vi "Climb.vi"(0 "Winch power":dbl=1.0, 1 "Toggle pistons":bool, 2 "Winch":bool, 3 "Unwinch":bool) -> ()   [LabVIEW 2019]
uses:
  <vilib>/Rock Robotics/WPI/Solenoid/WPI_SolenoidValue.ctl
  <vilib>/Rock Robotics/WPI/ThirdParty/Phoenix-LabVIEW/Motor Controller/Controls/CTRE_Phoenix_MotorControl_ControlMode.ctl
  <vilib>/functionblocks/FB Core/FB Core.xnode
  <vilib>/Rock Robotics/WPI/ThirdParty/Phoenix-LabVIEW/Motor Controller/Get/CTRE_Phoenix_MotorController_GetSupplyAndStatorCurrent_Enhanced.vi
  <vilib>/Rock Robotics/WPI/Solenoid/WPI_SolenoidSetEnum.vi
panel:
  out "Supply Current":dbl
  in  "Winch current threshold":dbl
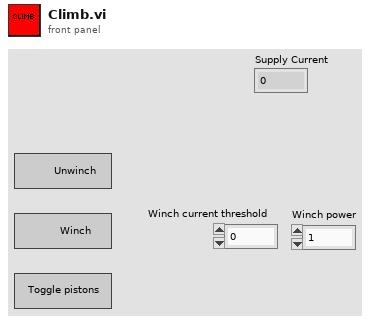
[diagram p1: front panel]
types:
  T1 = typedef "WPI_SolenoidValue.ctl" = enum16{"Off", "On", "Forward", "Reverse"}
  T2 = typedef "CTRE_Phoenix_MotorControl_ControlMode.ctl" = u16
  T3 = typedef "WPI_MotorControlDeviceRef.ctl" = cluster{"DeviceStatus":errorcluster, "Type":T4, "PWM":cluster{"PWM Channel":T5, "DeadBand":T6}, "CAN":cluster{"Device Number":u8, "SetOutput VI Ref":variant, "GetOutput VI Ref":variant, "Enable VI Ref":variant, "Disable VI Ref":variant, "Data":variant}, "Invert":bool, "DIO PWM":cluster{"PWM \"Enable\" Channel":T5, "DIOChannel":T7, "PWM Rate":dbl}}
  T4 = typedef "WPI_MotorControlType.ctl" = enum16{"PWM", "CAN", "DIO PWM"}
  T5 = typedef "FPGA_DIOPWMChannel.ctl" = enum8{"PWM 0", "PWM 1", "PWM 2", "PWM 3", "PWM 4", "PWM 5", "PWM 6", "PWM 7", "PWM 8", "PWM 9", "PWM MXP 0", "PWM MXP 1", "PWM MXP 2", "PWM MXP 3", "PWM MXP 4", "PWM MXP 5", "PWM MXP 6", "PWM MXP 7", "PWM MXP 8", "PWM MXP 9", "Invalid"}
  T6 = typedef "WPI_PWMDeadband.ctl" = cluster{"Name":string, "maxPositivePwm":i32, "minPositivePwm":i32, "centerPwm":i32, "maxNegativePwm":i32, "minNegativePwm":i32, "angularRange":u16}
  T7 = typedef "FPGA_DIOChannel.ctl" = enum8{"DIO 0", "DIO 1", "DIO 2", "DIO 3", "DIO 4", "DIO 5", "DIO 6", "DIO 7", "DIO 8", "DIO 9", "DIO MXP 0", "DIO MXP 1", "DIO MXP 2", "DIO MXP 3", "DIO MXP 4", "DIO MXP 5", "DIO MXP 6", "DIO MXP 7", "DIO MXP 8", "DIO MXP 9", "DIO MXP 10", "DIO MXP 11", "DIO MXP 12", "DIO MXP 13", "DIO MXP 14", "DIO MXP 15", "SPI Port CS1", "SPI Port CS2", "SPI Port CS3", "SPI Port MISO", "SPI Port MOSI", "Invalid"}
  T8 = typedef "WPI_SolenoidDevRef.ctl" = cluster{"DevStatus":errorcluster, "Pneumatics Control Module":u8, "Forward Solenoid Channel":T9, "Reverse Solenoid Channel":T9}
  T9 = typedef "WPI_SolenoidChannel.ctl" = enum8{"Solenoid 0", "Solenoid 1", "Solenoid 2", "Solenoid 3", "Solenoid 4", "Solenoid 5", "Solenoid 6", "Solenoid 7", "Invalid"}
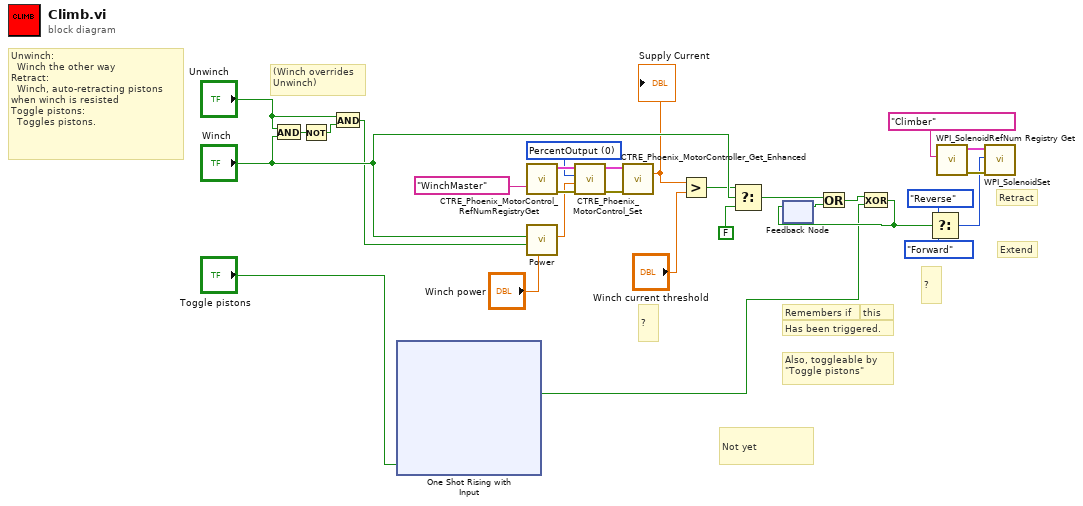
[diagram p0: block diagram]
diagram:
  w22 = T2 0 items=["PercentOutput"=0, "Position"=1, "Velocity"=2, "Current"=3, "Follower"=5, "MotionProfile"=6, "MotionMagic"=7, "MotionProfileArc"=10, "Disabled"=15] ("Control Mode")
  # "Extend"
  # "Retract"
  # "Not yet"
  # "Also, toggleable by \"Toggle pistons\""
  # "Has been triggered."
  # "this"
  # "Remembers if"
  # "?"
  # "?"
  # "(Winch overrides Unwinch)"
  # "Unwinch:\n  Winch the other way\nRetract:\n  Winch, auto-retracting pistons when winch is resisted\nToggle pistons:\n  Toggles pistons."
  n1 = And(x="Unwinch", y="Winch") -> (x .and. y?=w5:bool)
  n2 = Not(x=w5) -> (.not. x?=w6:bool)
  n3 = And(x="Unwinch", y=w6) -> (x .and. y?=w4:bool)
  n4 = xnode "One Shot Rising with Input"("input"="Toggle pistons") -> ("output"=w1:bool)  [unwired: 1 in, 1 out]
  n5 = call <vilib>:"CTRE_Phoenix_MotorControl_RefNumRegistryGet.vi"("refnum name"="WinchMaster") -> ("error out"=w19:errorcluster, "PhoenixMotorControlDevRef"=w23:T3)  [unwired: 9 in]
  n6 = call "Power.vi"("Positive Power"="Winch power", "Negative"=w4, "Positive"="Winch") -> ("Output"=w11:dbl)  [unwired: 8 in]
  n7 = call <vilib>:"CTRE_Phoenix_MotorControl_Set.vi"("error in (no error)"=w19, "Output"=w11, "Control Mode"=w22, "PhoenixMotorControlDevRef"=w23) -> ("error out"=w20:errorcluster, "PhoenixMotorControlDevRef"=w21:T3)  [unwired: 6 in]
  n8 = call-poly <vilib>:"CTRE_Phoenix_MotorController_Get_Enhanced.vi"("PhoenixMotorControlDevRef"=w21, "error in"=w20) -> ("Supply Current"=w17:dbl)  [unwired: 10 in, 3 out]
  "Supply Current" <- w17
  n9 = Greater?(x=w17, y="Winch current threshold") -> (0:w9:bool)
  n10 = Select(t=w9, s="Winch", f=FALSE) -> (s? t:f=w7:bool)
  n11 = feedback #1() -> (w12:bool)  [unwired: 1 in]
  n12 = Or(x=w7, y=w12) -> (x .or. y?=w3:bool)
  n13 = Exclusive Or(1:w1, 2:w3) -> (0:w2:bool)
  n14 = feedback-in #1(w2) -> ()
  n15 = Select(t=WPI_SolenoidValue."Reverse" ("Value"), s=w2, f=WPI_SolenoidValue."Forward" ("Value")) -> (s? t:f=w13:T1)
  n16 = call <vilib>:"WPI_SolenoidRefNum Registry Get.vi"("refnum name"="Climber") -> ("error out"=w18:errorcluster, "SolenoidDevRef"=w26:T8)  [unwired: 9 in]
  n17 = call-poly <vilib>:"WPI_SolenoidSet.vi"("error in (no error)"=w18, "Value"=w13, "SolenoidDevRef"=w26) -> ()  [unwired: 7 in, 2 out]
